vi "Read Axial Push Pressure.vi"(8 "error in (no error)":errorcluster, 11 "Model in":refnum<class "Model.lvclass">) -> (0 "error out":errorcluster, 3 "Model out":refnum<class "Model.lvclass">)   [LabVIEW 2015, in "Model.lvclass"]
uses:
  Model.lvclass
  Model.lvclass/Model.ctl
  DAQmx/DAQmx.lvclass
  Calculators/Volts To Pressure/Voltage To Pressure.lvclass
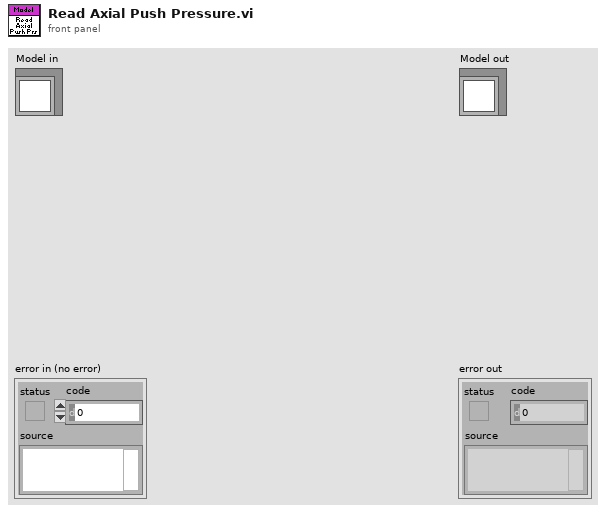
[diagram p1: front panel]
types:
  T1 = typedef "FAMT Typedefs.lvlib/Pressure Sensor Settings.ctl" = cluster{"Read Pressures":bool, "PSI per Volt":dbl, "Offset":dbl}
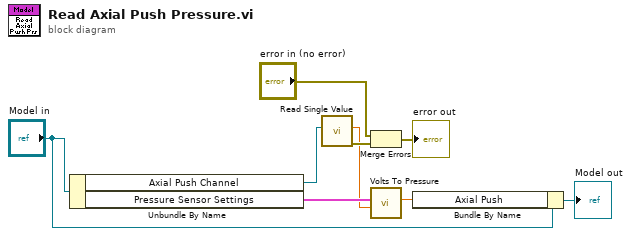
[diagram p0: block diagram]
diagram:
  n1 = Unbundle By Name("Model in") -> ("Axial Push Channel"=w9:refnum<k21>, "Pressure Sensor Settings"=w3:T1)
  n2 = call "Read Single Value.vi"("Channel"=w9) -> ("error out"=w7:errorcluster, "Value"=w2:dbl)  [unwired: 8 in, 1 out]
  n3 = Merge Errors("error in (no error)", w7) -> (→"error out":errorcluster)
  n4 = call "Volts To Pressure.vi"("Volts"=w2, "Pressure Sensor Settings"=w3) -> ("Pressure"=w1:dbl)  [unwired: 7 in, 2 out]
  n5 = Bundle By Name(cluster="Model in", "Axial Push"=w1) -> (→"Model out":refnum<class "Model.lvclass">)
